vi "Шифратор для клавиатуры.vi"(0 "Keyboard":T2) -> (1 "Bin":T1, 2 "cinp":bool)   [LabVIEW 2013]
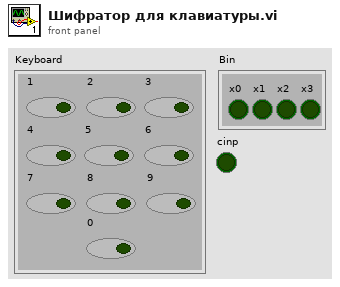
[diagram p1: front panel]
types:
  T1 = cluster{"x0":bool, "x1":bool, "x2":bool, "x3":bool}
  T2 = cluster{"0":bool, "1":bool, "2":bool, "3":bool, "4":bool, "5":bool, "6":bool, "7":bool, "8":bool, "9":bool}
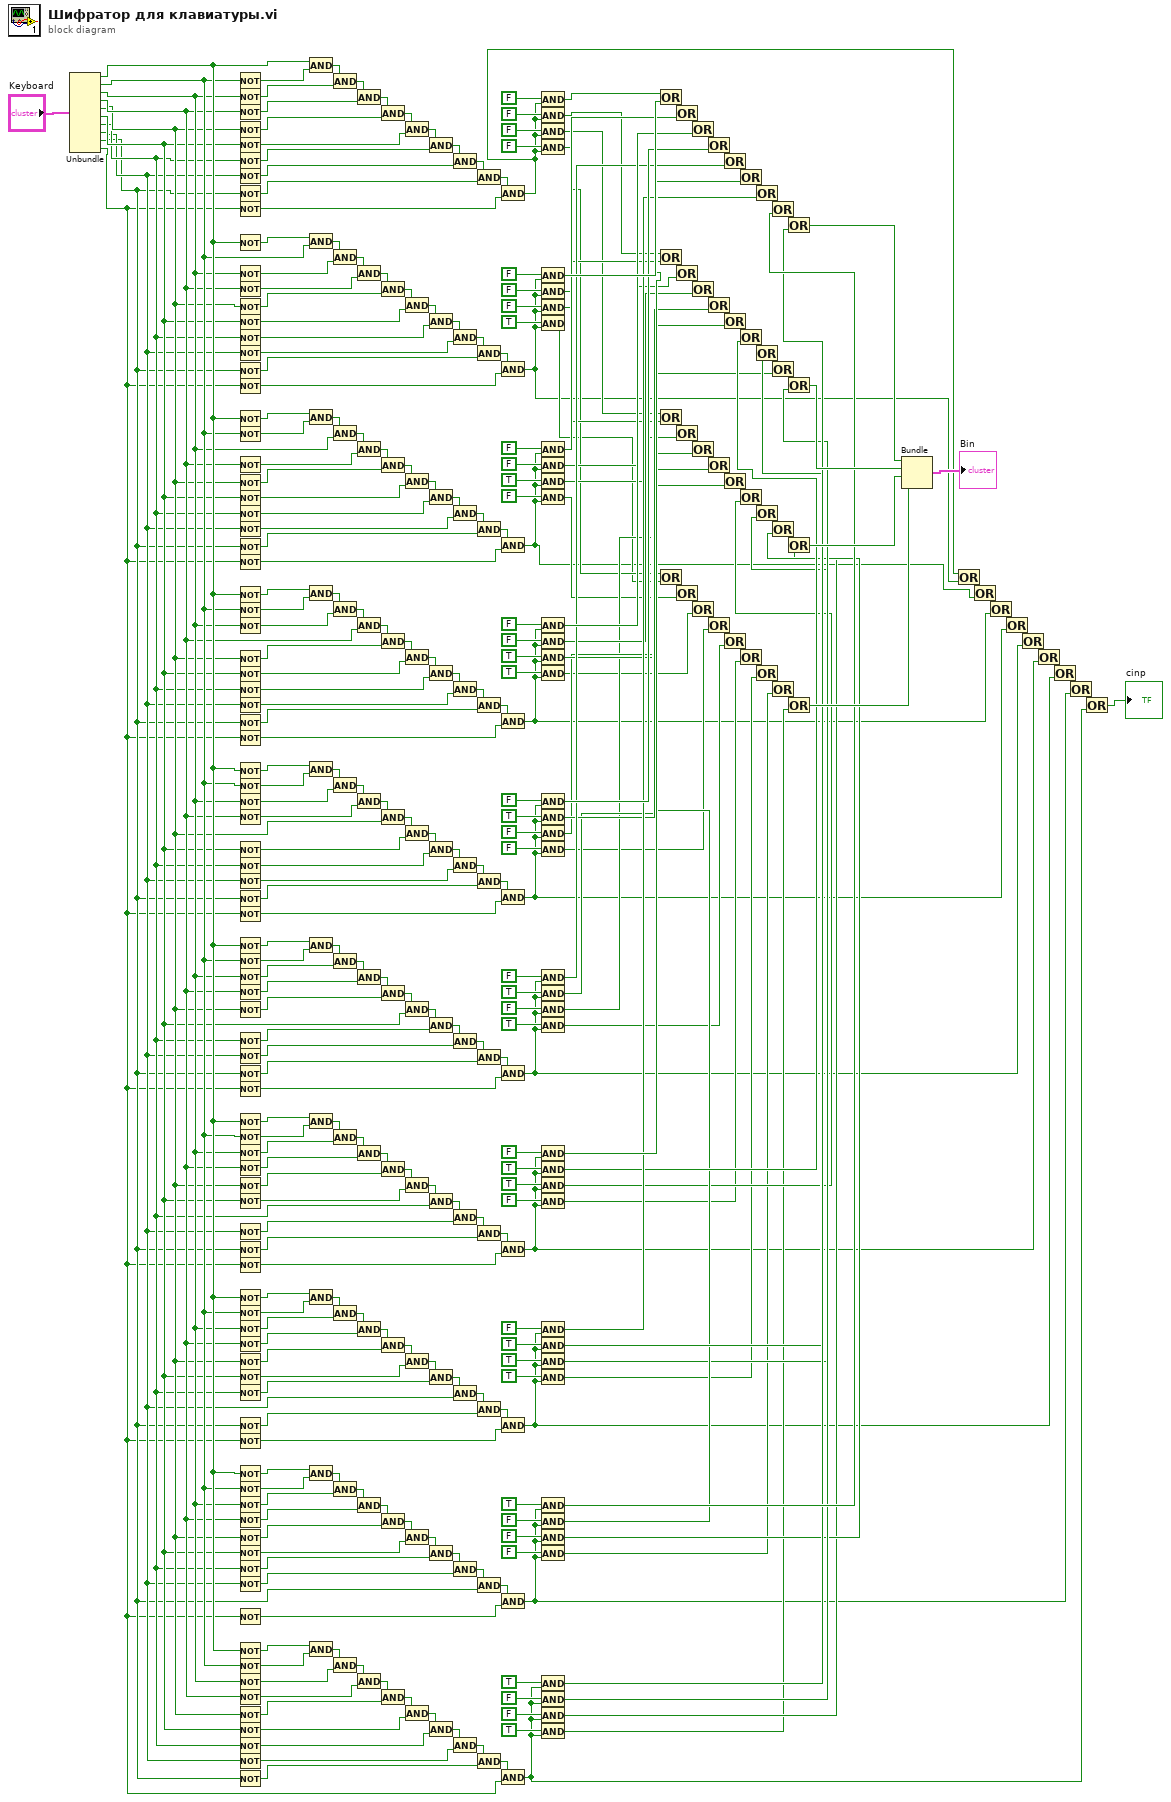
[diagram p0: block diagram]
diagram:
  n1 = Unbundle("Keyboard") -> ("0"=w29:bool, "1"=w28:bool, "2"=w27:bool, "3"=w26:bool, "4"=w25:bool, "5"=w24:bool, "6"=w23:bool, "7"=w22:bool, "8"=w21:bool, "9"=w20:bool)
  n2 = Not(x=w28) -> (.not. x?=w236:bool)
  n3 = Not(x=w27) -> (.not. x?=w235:bool)
  n4 = Not(x=w26) -> (.not. x?=w234:bool)
  n5 = Not(x=w25) -> (.not. x?=w233:bool)
  n6 = Not(x=w24) -> (.not. x?=w232:bool)
  n7 = Not(x=w23) -> (.not. x?=w231:bool)
  n8 = Not(x=w22) -> (.not. x?=w230:bool)
  n9 = Not(x=w21) -> (.not. x?=w229:bool)
  n10 = Not(x=w20) -> (.not. x?=w228:bool)
  n11 = Not(x=w29) -> (.not. x?=w227:bool)
  n12 = Not(x=w27) -> (.not. x?=w226:bool)
  n13 = Not(x=w26) -> (.not. x?=w225:bool)
  n14 = Not(x=w25) -> (.not. x?=w224:bool)
  n15 = Not(x=w24) -> (.not. x?=w223:bool)
  n16 = Not(x=w23) -> (.not. x?=w222:bool)
  n17 = Not(x=w22) -> (.not. x?=w221:bool)
  n18 = Not(x=w21) -> (.not. x?=w220:bool)
  n19 = Not(x=w20) -> (.not. x?=w219:bool)
  n20 = Not(x=w29) -> (.not. x?=w218:bool)
  n21 = Not(x=w28) -> (.not. x?=w217:bool)
  n22 = Not(x=w26) -> (.not. x?=w216:bool)
  n23 = Not(x=w25) -> (.not. x?=w215:bool)
  n24 = Not(x=w24) -> (.not. x?=w214:bool)
  n25 = Not(x=w23) -> (.not. x?=w213:bool)
  n26 = Not(x=w22) -> (.not. x?=w212:bool)
  n27 = Not(x=w21) -> (.not. x?=w211:bool)
  n28 = Not(x=w20) -> (.not. x?=w210:bool)
  n29 = Not(x=w29) -> (.not. x?=w209:bool)
  n30 = Not(x=w28) -> (.not. x?=w208:bool)
  n31 = Not(x=w27) -> (.not. x?=w207:bool)
  n32 = Not(x=w25) -> (.not. x?=w206:bool)
  n33 = Not(x=w24) -> (.not. x?=w205:bool)
  n34 = Not(x=w23) -> (.not. x?=w204:bool)
  n35 = Not(x=w22) -> (.not. x?=w203:bool)
  n36 = Not(x=w21) -> (.not. x?=w202:bool)
  n37 = Not(x=w20) -> (.not. x?=w201:bool)
  n38 = Not(x=w29) -> (.not. x?=w200:bool)
  n39 = Not(x=w28) -> (.not. x?=w199:bool)
  n40 = Not(x=w27) -> (.not. x?=w198:bool)
  n41 = Not(x=w26) -> (.not. x?=w197:bool)
  n42 = Not(x=w24) -> (.not. x?=w196:bool)
  n43 = Not(x=w23) -> (.not. x?=w195:bool)
  n44 = Not(x=w22) -> (.not. x?=w194:bool)
  n45 = Not(x=w21) -> (.not. x?=w193:bool)
  n46 = Not(x=w20) -> (.not. x?=w192:bool)
  n47 = Not(x=w29) -> (.not. x?=w191:bool)
  n48 = Not(x=w28) -> (.not. x?=w190:bool)
  n49 = Not(x=w27) -> (.not. x?=w189:bool)
  n50 = Not(x=w26) -> (.not. x?=w188:bool)
  n51 = Not(x=w25) -> (.not. x?=w187:bool)
  n52 = Not(x=w23) -> (.not. x?=w186:bool)
  n53 = Not(x=w22) -> (.not. x?=w185:bool)
  n54 = Not(x=w21) -> (.not. x?=w184:bool)
  n55 = Not(x=w20) -> (.not. x?=w183:bool)
  n56 = Not(x=w29) -> (.not. x?=w182:bool)
  n57 = Not(x=w28) -> (.not. x?=w181:bool)
  n58 = Not(x=w27) -> (.not. x?=w180:bool)
  n59 = Not(x=w26) -> (.not. x?=w179:bool)
  n60 = Not(x=w25) -> (.not. x?=w178:bool)
  n61 = Not(x=w24) -> (.not. x?=w177:bool)
  n62 = Not(x=w22) -> (.not. x?=w176:bool)
  n63 = Not(x=w21) -> (.not. x?=w175:bool)
  n64 = Not(x=w20) -> (.not. x?=w174:bool)
  n65 = Not(x=w29) -> (.not. x?=w173:bool)
  n66 = Not(x=w28) -> (.not. x?=w172:bool)
  n67 = Not(x=w27) -> (.not. x?=w171:bool)
  n68 = Not(x=w26) -> (.not. x?=w170:bool)
  n69 = Not(x=w25) -> (.not. x?=w169:bool)
  n70 = Not(x=w24) -> (.not. x?=w168:bool)
  n71 = Not(x=w23) -> (.not. x?=w167:bool)
  n72 = Not(x=w21) -> (.not. x?=w166:bool)
  n73 = Not(x=w20) -> (.not. x?=w165:bool)
  n74 = Not(x=w29) -> (.not. x?=w164:bool)
  n75 = Not(x=w28) -> (.not. x?=w163:bool)
  n76 = Not(x=w27) -> (.not. x?=w162:bool)
  n77 = Not(x=w26) -> (.not. x?=w161:bool)
  n78 = Not(x=w25) -> (.not. x?=w160:bool)
  n79 = Not(x=w24) -> (.not. x?=w159:bool)
  n80 = Not(x=w23) -> (.not. x?=w158:bool)
  n81 = Not(x=w22) -> (.not. x?=w157:bool)
  n82 = Not(x=w20) -> (.not. x?=w156:bool)
  n83 = Not(x=w29) -> (.not. x?=w155:bool)
  n84 = Not(x=w28) -> (.not. x?=w154:bool)
  n85 = Not(x=w27) -> (.not. x?=w153:bool)
  n86 = Not(x=w26) -> (.not. x?=w152:bool)
  n87 = Not(x=w25) -> (.not. x?=w151:bool)
  n88 = Not(x=w24) -> (.not. x?=w150:bool)
  n89 = Not(x=w23) -> (.not. x?=w149:bool)
  n90 = Not(x=w22) -> (.not. x?=w148:bool)
  n91 = Not(x=w21) -> (.not. x?=w147:bool)
  n92 = And(x=w29, y=w236) -> (x .and. y?=w316:bool)
  n93 = And(x=w227, y=w28) -> (x .and. y?=w308:bool)
  n94 = And(x=w218, y=w217) -> (x .and. y?=w300:bool)
  n95 = And(x=w209, y=w208) -> (x .and. y?=w292:bool)
  n96 = And(x=w200, y=w199) -> (x .and. y?=w284:bool)
  n97 = And(x=w191, y=w190) -> (x .and. y?=w276:bool)
  n98 = And(x=w182, y=w181) -> (x .and. y?=w268:bool)
  n99 = And(x=w173, y=w172) -> (x .and. y?=w260:bool)
  n100 = And(x=w164, y=w163) -> (x .and. y?=w252:bool)
  n101 = And(x=w155, y=w154) -> (x .and. y?=w244:bool)
  n102 = And(x=w316, y=w235) -> (x .and. y?=w315:bool)
  n103 = And(x=w308, y=w226) -> (x .and. y?=w307:bool)
  n104 = And(x=w300, y=w27) -> (x .and. y?=w299:bool)
  n105 = And(x=w292, y=w207) -> (x .and. y?=w291:bool)
  n106 = And(x=w284, y=w198) -> (x .and. y?=w283:bool)
  n107 = And(x=w276, y=w189) -> (x .and. y?=w275:bool)
  n108 = And(x=w268, y=w180) -> (x .and. y?=w267:bool)
  n109 = And(x=w260, y=w171) -> (x .and. y?=w259:bool)
  n110 = And(x=w252, y=w162) -> (x .and. y?=w251:bool)
  n111 = And(x=w244, y=w153) -> (x .and. y?=w243:bool)
  n112 = And(x=w315, y=w234) -> (x .and. y?=w314:bool)
  n113 = And(x=w307, y=w225) -> (x .and. y?=w306:bool)
  n114 = And(x=w299, y=w216) -> (x .and. y?=w298:bool)
  n115 = And(x=w291, y=w26) -> (x .and. y?=w290:bool)
  n116 = And(x=w283, y=w197) -> (x .and. y?=w282:bool)
  n117 = And(x=w275, y=w188) -> (x .and. y?=w274:bool)
  n118 = And(x=w267, y=w179) -> (x .and. y?=w266:bool)
  n119 = And(x=w259, y=w170) -> (x .and. y?=w258:bool)
  n120 = And(x=w251, y=w161) -> (x .and. y?=w250:bool)
  n121 = And(x=w243, y=w152) -> (x .and. y?=w242:bool)
  n122 = And(x=w314, y=w233) -> (x .and. y?=w313:bool)
  n123 = And(x=w306, y=w224) -> (x .and. y?=w305:bool)
  n124 = And(x=w298, y=w215) -> (x .and. y?=w297:bool)
  n125 = And(x=w290, y=w206) -> (x .and. y?=w289:bool)
  n126 = And(x=w282, y=w25) -> (x .and. y?=w281:bool)
  n127 = And(x=w274, y=w187) -> (x .and. y?=w273:bool)
  n128 = And(x=w266, y=w178) -> (x .and. y?=w265:bool)
  n129 = And(x=w258, y=w169) -> (x .and. y?=w257:bool)
  n130 = And(x=w250, y=w160) -> (x .and. y?=w249:bool)
  n131 = And(x=w242, y=w151) -> (x .and. y?=w241:bool)
  n132 = And(x=w313, y=w232) -> (x .and. y?=w312:bool)
  n133 = And(x=w305, y=w223) -> (x .and. y?=w304:bool)
  n134 = And(x=w297, y=w214) -> (x .and. y?=w296:bool)
  n135 = And(x=w289, y=w205) -> (x .and. y?=w288:bool)
  n136 = And(x=w281, y=w196) -> (x .and. y?=w280:bool)
  n137 = And(x=w273, y=w24) -> (x .and. y?=w272:bool)
  n138 = And(x=w265, y=w177) -> (x .and. y?=w264:bool)
  n139 = And(x=w257, y=w168) -> (x .and. y?=w256:bool)
  n140 = And(x=w249, y=w159) -> (x .and. y?=w248:bool)
  n141 = And(x=w241, y=w150) -> (x .and. y?=w240:bool)
  n142 = And(x=w312, y=w231) -> (x .and. y?=w311:bool)
  n143 = And(x=w304, y=w222) -> (x .and. y?=w303:bool)
  n144 = And(x=w296, y=w213) -> (x .and. y?=w295:bool)
  n145 = And(x=w288, y=w204) -> (x .and. y?=w287:bool)
  n146 = And(x=w280, y=w195) -> (x .and. y?=w279:bool)
  n147 = And(x=w272, y=w186) -> (x .and. y?=w271:bool)
  n148 = And(x=w264, y=w23) -> (x .and. y?=w263:bool)
  n149 = And(x=w256, y=w167) -> (x .and. y?=w255:bool)
  n150 = And(x=w248, y=w158) -> (x .and. y?=w247:bool)
  n151 = And(x=w240, y=w149) -> (x .and. y?=w239:bool)
  n152 = And(x=w311, y=w230) -> (x .and. y?=w310:bool)
  n153 = And(x=w303, y=w221) -> (x .and. y?=w302:bool)
  n154 = And(x=w295, y=w212) -> (x .and. y?=w294:bool)
  n155 = And(x=w287, y=w203) -> (x .and. y?=w286:bool)
  n156 = And(x=w279, y=w194) -> (x .and. y?=w278:bool)
  n157 = And(x=w271, y=w185) -> (x .and. y?=w270:bool)
  n158 = And(x=w263, y=w176) -> (x .and. y?=w262:bool)
  n159 = And(x=w255, y=w22) -> (x .and. y?=w254:bool)
  n160 = And(x=w247, y=w157) -> (x .and. y?=w246:bool)
  n161 = And(x=w239, y=w148) -> (x .and. y?=w238:bool)
  n162 = And(x=w310, y=w229) -> (x .and. y?=w309:bool)
  n163 = And(x=w302, y=w220) -> (x .and. y?=w301:bool)
  n164 = And(x=w294, y=w211) -> (x .and. y?=w293:bool)
  n165 = And(x=w286, y=w202) -> (x .and. y?=w285:bool)
  n166 = And(x=w278, y=w193) -> (x .and. y?=w277:bool)
  n167 = And(x=w270, y=w184) -> (x .and. y?=w269:bool)
  n168 = And(x=w262, y=w175) -> (x .and. y?=w261:bool)
  n169 = And(x=w254, y=w166) -> (x .and. y?=w253:bool)
  n170 = And(x=w246, y=w21) -> (x .and. y?=w245:bool)
  n171 = And(x=w238, y=w147) -> (x .and. y?=w237:bool)
  n172 = And(x=w309, y=w228) -> (x .and. y?=w10:bool)
  n173 = And(x=w301, y=w219) -> (x .and. y?=w9:bool)
  n174 = And(x=w293, y=w210) -> (x .and. y?=w8:bool)
  n175 = And(x=w285, y=w201) -> (x .and. y?=w7:bool)
  n176 = And(x=w277, y=w192) -> (x .and. y?=w6:bool)
  n177 = And(x=w269, y=w183) -> (x .and. y?=w5:bool)
  n178 = And(x=w261, y=w174) -> (x .and. y?=w4:bool)
  n179 = And(x=w253, y=w165) -> (x .and. y?=w3:bool)
  n180 = And(x=w245, y=w156) -> (x .and. y?=w2:bool)
  n181 = And(x=w237, y=w20) -> (x .and. y?=w1:bool)
  n182 = And(x=FALSE, y=w10) -> (x .and. y?=w69:bool)
  n183 = And(x=FALSE, y=w10) -> (x .and. y?=w59:bool)
  n184 = And(x=FALSE, y=w10) -> (x .and. y?=w49:bool)
  n185 = And(x=FALSE, y=w10) -> (x .and. y?=w39:bool)
  n186 = And(x=FALSE, y=w9) -> (x .and. y?=w68:bool)
  n187 = And(x=FALSE, y=w9) -> (x .and. y?=w58:bool)
  n188 = And(x=FALSE, y=w9) -> (x .and. y?=w48:bool)
  n189 = And(x=TRUE, y=w9) -> (x .and. y?=w38:bool)
  n190 = And(x=FALSE, y=w8) -> (x .and. y?=w67:bool)
  n191 = And(x=FALSE, y=w8) -> (x .and. y?=w57:bool)
  n192 = And(x=TRUE, y=w8) -> (x .and. y?=w47:bool)
  n193 = And(x=FALSE, y=w8) -> (x .and. y?=w37:bool)
  n194 = And(x=FALSE, y=w7) -> (x .and. y?=w66:bool)
  n195 = And(x=FALSE, y=w7) -> (x .and. y?=w56:bool)
  n196 = And(x=TRUE, y=w7) -> (x .and. y?=w46:bool)
  n197 = And(x=TRUE, y=w7) -> (x .and. y?=w36:bool)
  n198 = And(x=FALSE, y=w6) -> (x .and. y?=w65:bool)
  n199 = And(x=TRUE, y=w6) -> (x .and. y?=w55:bool)
  n200 = And(x=FALSE, y=w6) -> (x .and. y?=w45:bool)
  n201 = And(x=FALSE, y=w6) -> (x .and. y?=w35:bool)
  n202 = And(x=FALSE, y=w5) -> (x .and. y?=w64:bool)
  n203 = And(x=TRUE, y=w5) -> (x .and. y?=w54:bool)
  n204 = And(x=FALSE, y=w5) -> (x .and. y?=w44:bool)
  n205 = And(x=TRUE, y=w5) -> (x .and. y?=w34:bool)
  n206 = And(x=FALSE, y=w4) -> (x .and. y?=w63:bool)
  n207 = And(x=TRUE, y=w4) -> (x .and. y?=w53:bool)
  n208 = And(x=TRUE, y=w4) -> (x .and. y?=w43:bool)
  n209 = And(x=FALSE, y=w4) -> (x .and. y?=w33:bool)
  n210 = And(x=FALSE, y=w3) -> (x .and. y?=w62:bool)
  n211 = And(x=TRUE, y=w3) -> (x .and. y?=w52:bool)
  n212 = And(x=TRUE, y=w3) -> (x .and. y?=w42:bool)
  n213 = And(x=TRUE, y=w3) -> (x .and. y?=w32:bool)
  n214 = And(x=TRUE, y=w2) -> (x .and. y?=w61:bool)
  n215 = And(x=FALSE, y=w2) -> (x .and. y?=w51:bool)
  n216 = And(x=FALSE, y=w2) -> (x .and. y?=w41:bool)
  n217 = And(x=FALSE, y=w2) -> (x .and. y?=w31:bool)
  n218 = And(x=TRUE, y=w1) -> (x .and. y?=w60:bool)
  n219 = And(x=FALSE, y=w1) -> (x .and. y?=w50:bool)
  n220 = And(x=FALSE, y=w1) -> (x .and. y?=w40:bool)
  n221 = And(x=TRUE, y=w1) -> (x .and. y?=w30:bool)
  n222 = Or(x=w69, y=w68) -> (x .or. y?=w106:bool)
  n223 = Or(x=w59, y=w58) -> (x .or. y?=w98:bool)
  n224 = Or(x=w49, y=w48) -> (x .or. y?=w90:bool)
  n225 = Or(x=w39, y=w38) -> (x .or. y?=w82:bool)
  n226 = Or(x=w106, y=w67) -> (x .or. y?=w105:bool)
  n227 = Or(x=w98, y=w57) -> (x .or. y?=w97:bool)
  n228 = Or(x=w90, y=w47) -> (x .or. y?=w89:bool)
  n229 = Or(x=w82, y=w37) -> (x .or. y?=w81:bool)
  n230 = Or(x=w105, y=w66) -> (x .or. y?=w104:bool)
  n231 = Or(x=w97, y=w56) -> (x .or. y?=w96:bool)
  n232 = Or(x=w89, y=w46) -> (x .or. y?=w88:bool)
  n233 = Or(x=w81, y=w36) -> (x .or. y?=w80:bool)
  n234 = Or(x=w104, y=w65) -> (x .or. y?=w103:bool)
  n235 = Or(x=w96, y=w55) -> (x .or. y?=w95:bool)
  n236 = Or(x=w88, y=w45) -> (x .or. y?=w87:bool)
  n237 = Or(x=w80, y=w35) -> (x .or. y?=w79:bool)
  n238 = Or(x=w103, y=w64) -> (x .or. y?=w102:bool)
  n239 = Or(x=w95, y=w54) -> (x .or. y?=w94:bool)
  n240 = Or(x=w87, y=w44) -> (x .or. y?=w86:bool)
  n241 = Or(x=w79, y=w34) -> (x .or. y?=w78:bool)
  n242 = Or(x=w102, y=w63) -> (x .or. y?=w101:bool)
  n243 = Or(x=w94, y=w53) -> (x .or. y?=w93:bool)
  n244 = Or(x=w86, y=w43) -> (x .or. y?=w85:bool)
  n245 = Or(x=w78, y=w33) -> (x .or. y?=w77:bool)
  n246 = Or(x=w101, y=w62) -> (x .or. y?=w100:bool)
  n247 = Or(x=w93, y=w52) -> (x .or. y?=w92:bool)
  n248 = Or(x=w85, y=w42) -> (x .or. y?=w84:bool)
  n249 = Or(x=w77, y=w32) -> (x .or. y?=w76:bool)
  n250 = Or(x=w100, y=w61) -> (x .or. y?=w99:bool)
  n251 = Or(x=w92, y=w51) -> (x .or. y?=w91:bool)
  n252 = Or(x=w84, y=w41) -> (x .or. y?=w83:bool)
  n253 = Or(x=w76, y=w31) -> (x .or. y?=w75:bool)
  n254 = Or(x=w99, y=w60) -> (x .or. y?=w73:bool)
  n255 = Or(x=w91, y=w50) -> (x .or. y?=w72:bool)
  n256 = Or(x=w83, y=w40) -> (x .or. y?=w71:bool)
  n257 = Or(x=w75, y=w30) -> (x .or. y?=w70:bool)
  n258 = Bundle(w73, w72, w71, w70) -> (→"Bin":cluster{bool, bool, bool, bool})  [unwired: 1 in]
  n259 = Or(x=w10, y=w9) -> (x .or. y?=w19:bool)
  n260 = Or(x=w19, y=w8) -> (x .or. y?=w18:bool)
  n261 = Or(x=w18, y=w7) -> (x .or. y?=w17:bool)
  n262 = Or(x=w17, y=w6) -> (x .or. y?=w16:bool)
  n263 = Or(x=w16, y=w5) -> (x .or. y?=w15:bool)
  n264 = Or(x=w15, y=w4) -> (x .or. y?=w14:bool)
  n265 = Or(x=w14, y=w3) -> (x .or. y?=w13:bool)
  n266 = Or(x=w13, y=w2) -> (x .or. y?=w12:bool)
  n267 = Or(x=w12, y=w1) -> (x .or. y?=→"cinp":bool)
